vi "Refresh Feed (By Folder).vi"(8 "error in":errorcluster, 11 "feed folderpath in":path) -> (0 "error out":errorcluster, 3 "feed folderpath out":path)   [LabVIEW 2014, in "NIPM_API.lvlib"]
doc: "Refreshes NI Package Manager with data from a registered feed. \n\nNote: You should refresh after adding/removing packages from feeds, so that NI Package Manager will update with the latest feed and package data.\n\nINPUT(s)\n<B>Feed folderpath</B>: Specifies the folder containing the registered feed\n\nOUTPUT(s)\n<B>Feed folderpath out</B>: Outputs the specified feed folderpath"
uses:
  NIPM_API.lvlib
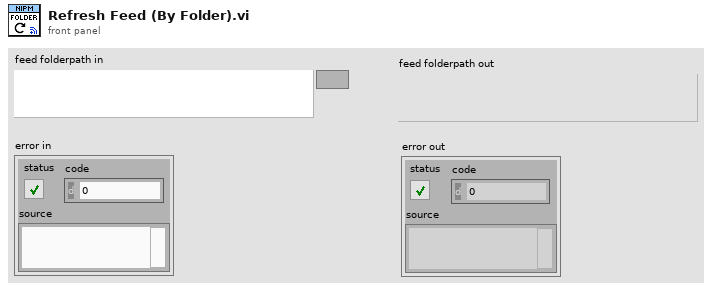
[diagram p1: front panel]
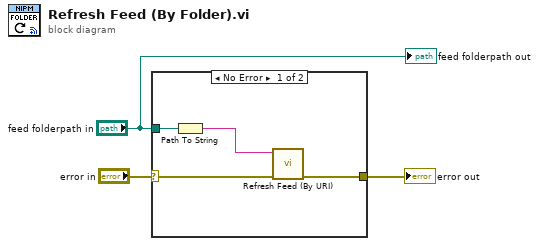
[diagram p0: block diagram]
diagram:
  n1 = case shown="No Error" "error in" {
    selector: "error in" -> [w7 w8]
    tunnel: [w4 w8] -> w2
    tunnel: "feed folderpath in" -> [w6 _]
    frame No Error {
      n2 = Path To String(path=w6) -> (string=w5:string)
      n3 = call "Refresh Feed (By URI).vi"("error in (no error)"=w7, "feed URI in"=w5) -> ("error out"=w4:errorcluster)  [unwired: 8 in, 1 out]
    }
    frame Error {
    }
  }
  "error out" <- w2
  "feed folderpath out" <- "feed folderpath in"
